vi "DBL Round.vi"(1 "반올림 옵션":enum16{"반올림", "올림", "내림"}(ring), 2 "반올림자리수":i32=1, 3 "DBL in":dbl format="%#_15g") -> (0 "DBL out":dbl format="%#_15g")   [LabVIEW 2020]
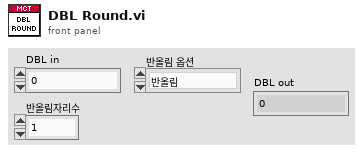
[diagram p1: front panel]
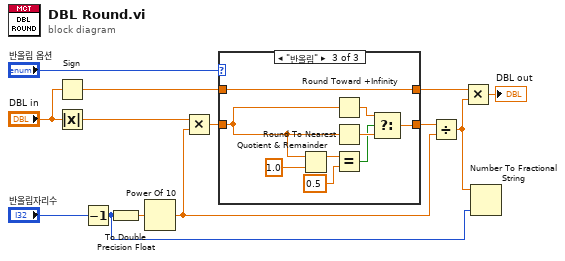
[diagram p0: block diagram]
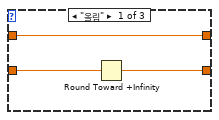
[diagram p2: hidden frame]
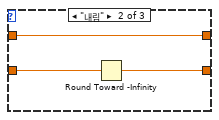
[diagram p3: hidden frame]
diagram:
  n1 = Sign(1:"DBL in") -> (0:w12:dbl)
  n2 = Absolute Value(x="DBL in") -> (abs(x)=w8:dbl)
  n3 = Decrement(x="반올림자리수") -> (x-1=w1:i32)
  n4 = To Double Precision Float(number=w1) -> (double precision float=w9:dbl)
  n5 = Power Of 10(x=w9) -> (10^x=w3:dbl)
  n6 = Multiply(x=w8, y=w3) -> (x*y=w7:dbl)
  n7 = case shown="\"반올림\"" "반올림 옵션" {
    tunnel: [w16 w18 w27] -> w6
    tunnel: w7 -> [w15 w19 w28]
    tunnel: w12 -> [w16 w18 w27]
    tunnel: [w14 w17 w20] -> w4
    frame "올림" {
      n8 = Round Toward +Infinity(x=w15) -> (ceil(x): smallest int >= x=w14:dbl)
    }
    frame "내림" {
      n9 = Round Toward -Infinity(1:w19) -> (0:w17:dbl)
    }
    frame "반올림" {
      n10 = Quotient & Remainder(x=w28, y=1.0) -> (x-y*floor(x/y)=w24:dbl)  [unwired: 1 out]
      n11 = Round Toward +Infinity(x=w28) -> (ceil(x): smallest int >= x=w26:dbl)
      n12 = Round To Nearest(number=w28) -> (nearest integer value=w25:dbl)
      n13 = Equal?(x=w24, y=0.5) -> (x = y?=w21:bool)
      n14 = Select(t=w26, s=w21, f=w25) -> (s? t:f=w20:dbl)
    }
  }
  n15 = Divide(x=w4, y=w3) -> (x/y=w2:dbl)
  n16 = Multiply(x=w6, y=w2) -> (x*y=→"DBL out":dbl)
  n17 = Number To Fractional String(number=w2, precision (6)=w1) -> ()  [unwired: 2 in, 1 out]
